vi "FPGA myRIOMain_v3.vi"() -> ()   [LabVIEW 2019]
doc: "Main FPGA VI\nUse the bitfile generated by this VI in the real-time code.\n\nFlip the channels for input and output"
uses:
  TypeDefs/AO mode TabCtrl.ctl
  TypeDefs/SamplingModeEnum.ctl
  <vilib>/rvi/Emulation/niFpgaGetClockAttributes.vi
  <vilib>/rvi/Emulation/niFpgaSctlEmulationGetInTimedLoop.vi
  <vilib>/rvi/Emulation/niFpgaEmulationReportErrorSimple.vi
  <vilib>/rvi/eio/common/nirviEmuTemplateMethod_errors.vi
  <vilib>/rvi/Emulation/niFpgaEmulationIsFPGAContextNoSignature.vi
  <vilib>/rvi/errors/niFpgaSetErrorForExecOnDevCompSimple.vi
  <vilib>/rvi/eio/common/nirviEmuReportErrorAndStop.vi
  <vilib>/rvi/DataTransferAndStorage/Container/Common/niFpgaContainerGetUniqueNameForEmu.vi
  <vilib>/rvi/FIFO/Fifo_Resource/nirvififoEmulationSetSize.vi
  <vilib>/rvi/FIFO/Fifo_Resource/nirviFifoEmulationQueueMgr.vi
  <instcachedir>/0/nirviFifoEmulationQueueMgr_E5CAEC123FF24DC58D834DCA3CDAA9B5.lvgen/nirviFifoEmulationQueueMgr_E5CAEC123FF24DC58D834DCA3CDAA9B5_003.vi
  <vilib>/rvi/FIFO/Fifo_Resource/nirvififoEmulationDetermineInputValidOut.vi
  <vilib>/rvi/FIFO/Fifo_Resource/nirvififoEmulationCreateLock.vi
  <vilib>/rvi/Emulation/niFpgaProcessEmulError.vi
  <vilib>/rvi/FIFO/Fifo_Resource/nirvififoEmulationObtainLock.vi
  <vilib>/rvi/FIFO/Fifo_Resource/nirvififoEmulationReleaseLock.vi
  <vilib>/rvi/occurrence/nirviWaitOnOccurrenceBase.vi
  <vilib>/rvi/errors/nirviReportUnexpectedCaseInternalError.vi
  <vilib>/rvi/errors/nirviReportUnexpectedCaseInternalError (U32).vi
  <vilib>/rvi/Emulation/niFpgaCriticalErrorInLSC.vi
  <vilib>/Utility/error.llb/Clear Errors.vi
  <vilib>/eio/EIONode/EIONode.xnode
  <vilib>/rvi/DataTransferAndStorage/Container/XNode/niFpgaContainer.xnode
  <vilib>/rvi/FIFO/Fifo_Resource/nirvififoEmulationWrite.vi
  <vilib>/rvi/FIFO/Fifo_Resource/nirvififoEmulationRead.vi
  <vilib>/rvi/Analysis/measure/butterworth/XNode/niFpgaButterworthFilter.xnode
  <vilib>/rvi/FXPMathLib/FxpMul/XNode/nifxpmath_Multiplier.xnode
  FPGA functions/FPGA functions.lvlib
  <vilib>/rvi/FXPMathLib/sim/FxpSim.dll
panel:
  out "Unable to\nrun at desired\nSample Time?":bool
  out "Processing Loop time [ticks]":u32
  out "FPGA AI DMA\nOverflow?":bool
  in  "Scaled Butterworth Coeffs":i32[](array[numeric])=[-1036986264, 2110353124, 93741, -1058362983, 2131726043, 94691]
  in  "Sampling Mode":T1
  in  "Bit-resolution":i8=12
  in  "AO mode":T2
  in  "AO Out [V]":fxp<+/-,18,5> format="%#.6g"
  in  "AO enable?":bool
  out "AI In [V]":fxp<+/-,25,5> format="%#.6g"
  out "FPGA AO DMA\nOverflow?":bool
  out "Int. Output":i16
  out "Raw Int. Input":i16
  in  "Sample Time [ticks]":u32=120
  out "AO Loop time [ticks]":u32
  out "AI Loop time [ticks]":u32
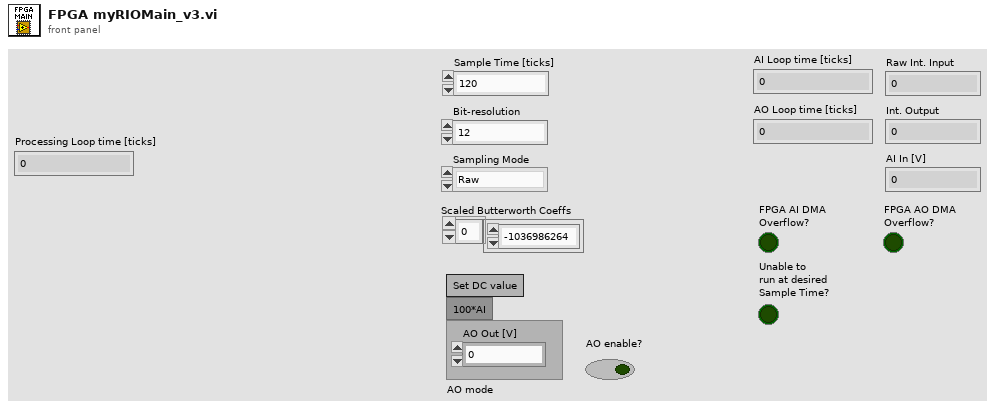
[diagram p1: front panel]
types:
  T1 = typedef "SamplingModeEnum.ctl" = enum16{"Raw", "LPF", "4 pt. Avg. + LPF"}
  T2 = typedef "AO mode TabCtrl.ctl" = enum32{"Set DC value", "100*AI"}
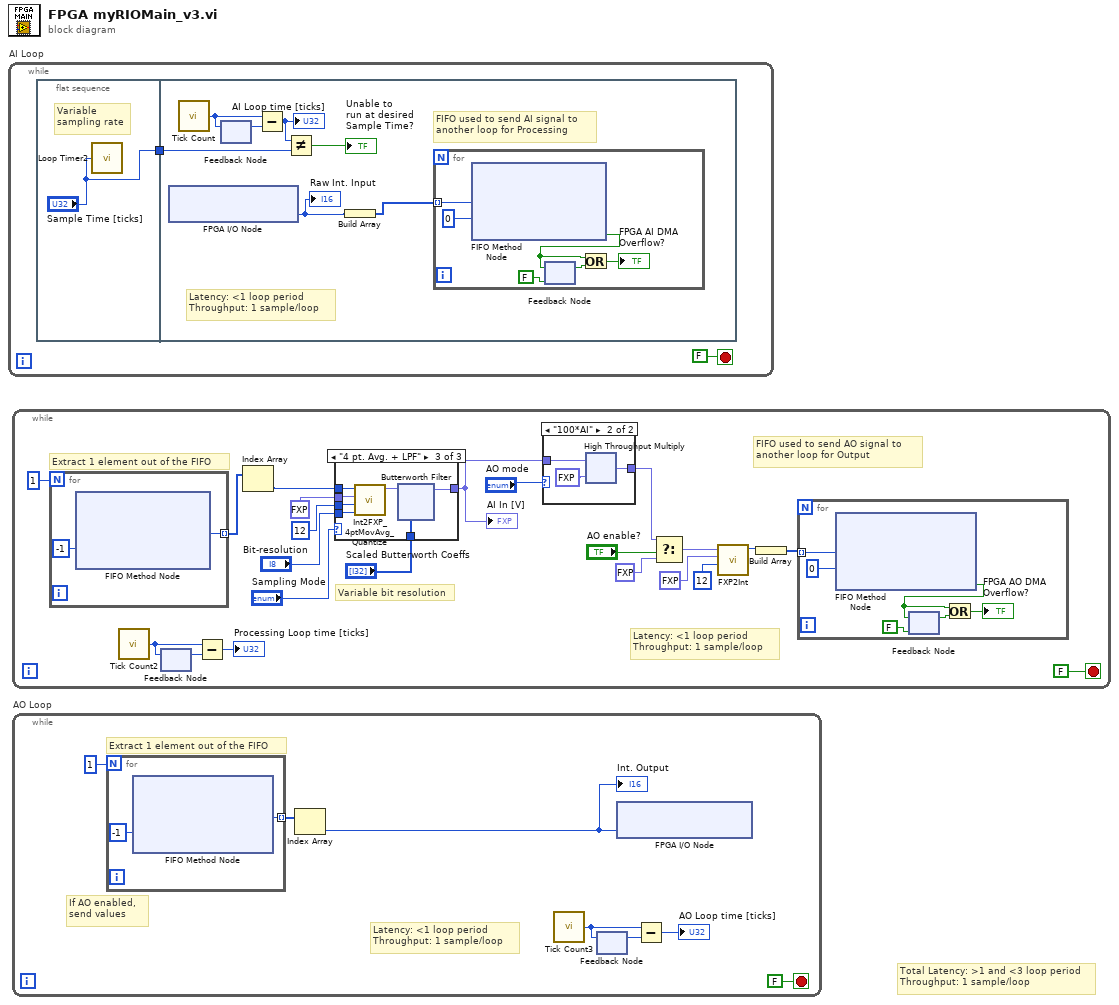
[diagram p0: block diagram]
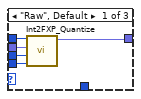
[diagram p2: hidden frame]
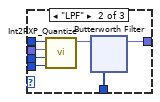
[diagram p3: hidden frame]
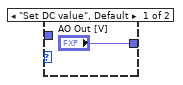
[diagram p4: hidden frame]
diagram:
  # "Total Latency: >1 and <3 loop period\nThroughput: 1 sample/loop"
  n1 = while "AI Loop" {
    stop <- FALSE stop-if-true
    n2 = flat-sequence {
      tunnel: ["Sample Time [ticks]"] -> w1
      tunnel: w1 -> [w5]
      frame #0 {
        # "Variable\nsampling rate"
        n3 = call "Loop Timer2"("Count(Ticks)"="Sample Time [ticks]") -> ()  [unwired: 1 out]
      }
      frame #1 {
        # "FIFO used to send AI signal to \nanother loop for Processing"
        # "Latency: <1 loop period\nThroughput: 1 sample/loop"
        n4 = xnode "FPGA I/O Node"() -> ("ConnectorC/AI0"=w8:i16)  [unwired: 1 in, 1 out]
        "Raw Int. Input" <- w8
        n5 = call "Tick Count"() -> ("Tick Count(Ticks)"=w10:u32)
        n6 = feedback #1() -> (w9:u32)  [unwired: 1 in]
        n7 = feedback-in #1(w10) -> ()
        n8 = Subtract(x=w10, y=w9) -> (x-y=w6:u32)
        "AI Loop time [ticks]" <- w6
        n9 = Not Equal?(x=w6, y=w5) -> (x != y?=→"Unable to\nrun at desired\nSample Time?":bool)
        n10 = Build Array(w8) -> (w7:i16[])
        n11 = for {
          tunnel: w7 -> [w13] mode=indexing
          n12 = xnode ("FIFO Method Node")("Element"=w13, "Timeout"=0) -> ("Timed Out?"=w11:bool)  [unwired: 1 in, 1 out]
          n13 = feedback-in #2(w11) -> ()
          n14 = feedback #2(FALSE ("Timed Out?")) -> (w15:bool)
          n15 = Or(x=w11, y=w15) -> (x .or. y?=→"FPGA AI DMA\nOverflow?":bool)
        }
      }
    }
  }
  n16 = while {
    stop <- FALSE stop-if-true
    # "Extract 1 element out of the FIFO"
    # "Variable bit resolution"
    # "Latency: <1 loop period\nThroughput: 1 sample/loop"
    # "FIFO used to send AO signal to \nanother loop for Output"
    n17 = for {
      N: 1 -> [_]
      tunnel: [w40] -> w21 mode=indexing
      n18 = xnode ("FIFO Method Node")("Timeout"=-1) -> ("Element"=w40:i16)  [unwired: 1 in, 2 out]
    }
    n19 = call "Tick Count2"() -> ("Tick Count(Ticks)"=w20:u32)
    n20 = feedback #3() -> (w19:u32)  [unwired: 1 in]
    n21 = feedback-in #3(w20) -> ()
    n22 = Subtract(x=w20, y=w19) -> (x-y=→"Processing Loop time [ticks]":u32)
    n23 = Index Array(array=w21) -> (element=w22:i16)  [unwired: 1 in]
    n24 = case shown="\"4 pt. Avg. + LPF\"" "Sampling Mode" {
      tunnel: i8 12 ("Input Bit resolution") -> [w45 w48 w66]
      tunnel: fxp<+,8,4> 10.0 ("Multiplier") -> [w44 w49 w67]
      tunnel: "Bit-resolution" -> [w43 w47 w65]
      tunnel: w22 -> [w42 w52 w63]
      tunnel: "Scaled Butterworth Coeffs" -> [_ w50 w62]
      tunnel: [w41 w46 w61] -> w24
      frame "Raw", Default {
        n25 = call "Int2FXP_Quantize.vi"("Output Bit resolution"=w43, "Input Bit resolution"=w45, "Multiplier"=w44, "Input (Int)"=w42) -> ("Output (FXP)"=w41:fxp<+/-,25,5>)  [unwired: 7 in]
      }
      frame "LPF" {
        n26 = call "Int2FXP_Quantize.vi"("Output Bit resolution"=w47, "Input Bit resolution"=w48, "Multiplier"=w49, "Input (Int)"=w52) -> ("Output (FXP)"=w51:fxp<+/-,25,5>)  [unwired: 7 in]
        n27 = xnode "Butterworth Filter"("input data"=w51, "scaled coefficients"=w50) -> ("output data"=w46:fxp<+/-,25,5>)  [unwired: 1 in]
      }
      frame "4 pt. Avg. + LPF" {
        n28 = call "Int2FXP_4ptMovAvg_Quantize.vi"("Output Bit resolution"=w65, "Input Bit resolution"=w66, "Multiplier"=w67, "Input (Int)"=w63) -> ("Output (FXP)"=w64:fxp<+/-,25,5>)  [unwired: 7 in]
        n29 = xnode "Butterworth Filter"("input data"=w64, "scaled coefficients"=w62) -> ("output data"=w61:fxp<+/-,25,5>)  [unwired: 1 in]
      }
    }
    "AI In [V]" <- w24
    n30 = case shown="\"100*AI\"" "AO mode" {
      tunnel: ["AO Out [V]" w77] -> w31
      tunnel: w24 -> [_ w79]
      frame "Set DC value", Default {
      }
      frame "100*AI" {
        n31 = xnode ("High Throughput Multiply")("x"=w79, "y"=fxp<+,5,7> 100.0) -> ("x*y"=w77:fxp<+/-,18,5>)
      }
    }
    n32 = Select(t=w31, s="AO enable?", f=fxp<+/-,18,5> 0.0) -> (s? t:f=w32:fxp<+/-,18,5>)
    n33 = call "FXP2Int.vi"("Output Bit resolution"=i8 12 ("Bit resolution"), "Multiplier"=fxp<+,18,-1> 0.10000038146972656, "Input (FXP)"=w32) -> ("Output (Int)"=w38:i16)  [unwired: 8 in]
    n34 = Build Array(w38) -> (w33:i16[])
    n35 = for {
      tunnel: w33 -> [w82] mode=indexing
      n36 = xnode ("FIFO Method Node")("Element"=w82, "Timeout"=0) -> ("Timed Out?"=w80:bool)  [unwired: 1 in, 1 out]
      n37 = feedback-in #4(w80) -> ()
      n38 = feedback #4(FALSE ("Timed Out?")) -> (w84:bool)
      n39 = Or(x=w80, y=w84) -> (x .or. y?=→"FPGA AO DMA\nOverflow?":bool)
    }
  }
  n40 = while "AO Loop" {
    stop <- FALSE stop-if-true
    # "Latency: <1 loop period\nThroughput: 1 sample/loop"
    # "If AO enabled, \nsend values"
    # "Extract 1 element out of the FIFO"
    n41 = for {
      N: 1 -> [_]
      tunnel: [w94] -> w88 mode=indexing
      n42 = xnode ("FIFO Method Node")("Timeout"=-1) -> ("Element"=w94:i16)  [unwired: 1 in, 2 out]
    }
    n43 = Index Array(array=w88) -> (element=w86:i16)  [unwired: 1 in]
    "Int. Output" <- w86
    n44 = call "Tick Count3"() -> ("Tick Count(Ticks)"=w91:u32)
    n45 = feedback #5() -> (w90:u32)  [unwired: 1 in]
    n46 = feedback-in #5(w91) -> ()
    n47 = xnode "FPGA I/O Node"("ConnectorC/AO0"=w86) -> ()  [unwired: 1 in, 1 out]
    n48 = Subtract(x=w91, y=w90) -> (x-y=→"AO Loop time [ticks]":u32)
  }
